vi "Library Absolve Path.vi"(0 "absolute base":path, 7 "input path to absolve":path) -> (8 "absolved path":path)   [LabVIEW 2012]
doc: "Takes an input path and ensures that it is resolved to an absolute path. If the input path is already absolute, it is left unchanged. If the input path is relative, the provided absolute base path is prepended. If the input path is empty, the provided absolute base path is returned."
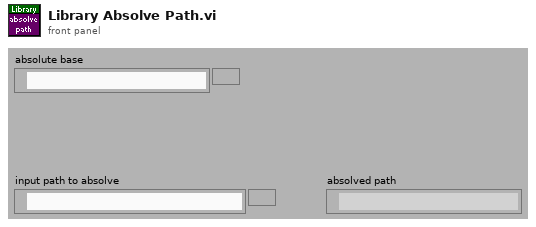
[diagram p1: front panel]
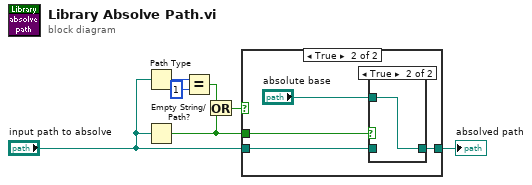
[diagram p0: block diagram]
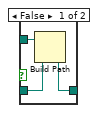
[diagram p3: hidden frame]
diagram:
  n1 = Path Type(1:"input path to absolve") -> (0:w1:i16)
  n2 = Empty String/Path?(string/path="input path to absolve") -> (empty?=w5:bool)
  n3 = Equal?(x=w1, y=i16 1) -> (x = y?=w4:bool)
  n4 = Or(x=w4, y=w5) -> (x .or. y?=w3:bool)
  n5 = case shown="True" w3 {
    tunnel: "input path to absolve" -> [w8 w12]
    tunnel: [w8 w11] -> w7
    tunnel: w5 -> [_ w10]
    frame False {
    }
    frame True {
      n6 = case shown="True" w10 {
        tunnel: "absolute base" -> [w15 w16]
        tunnel: w12 -> [w14 _]
        tunnel: [w13 w16] -> w11
        frame False {
          n7 = Build Path(base path=w15, name or relative path=w14) -> (appended path=w13:path)
        }
        frame True {
        }
      }
    }
  }
  "absolved path" <- w7
